vi "IsSatisfied.vi"(10 "Product":refnum<class "Product.lvclass">, 11 "IFilterSpecification":refnum<class "IFilterSpecification.lvclass">) -> (2 "IsSatisfied":bool)   [LabVIEW 2018, in "IFilterSpecification.lvclass"]
uses:
  IFilterSpecification/IFilterSpecification.lvclass
  Product/Product.lvclass
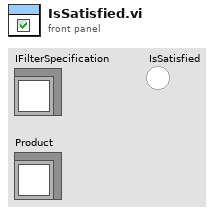
[diagram p1: front panel]
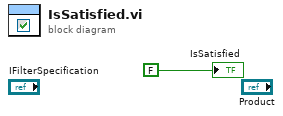
[diagram p0: block diagram]
diagram:
  "IsSatisfied" <- FALSE ("IsSatisfied")
